vi "Examples.vi"() -> ()   [LabVIEW 2019]
uses:
  <userlib>/MicroPython/VIs/uPythonX/uPythonX.xctl
panel:
  in  "Tab Control":enum32{"Simple", "Page 2"}(tab)
  in  "Driving":T1(xcontrol)={"Port"="130.64.157.92", "All Code"="#!/usr/bin/env pybricks-micropython\n\nfrom pybricks import ev3brick as brick\nfrom pybricks.ev3devices import (Motor, TouchSensor, \n          ColorSensor,InfraredSensor, UltrasonicSensor, GyroSensor)\nfrom pybricks.parameters import (Port, Stop, Direction, Button, Color,\n                                   SoundFile, ImageFile, Align)\nfrom pybricks.tools import print, wait, StopWatch\nfrom pybricks.robotics import DriveBase\nimport time\n\n# plug in\n# A =  left motor\n# D =  right motor\n# \n# S4 =  ultrasonic sensor\n\nleft = Motor(Port.A)\nright = Motor(Port.D)\ndist = UltrasonicSensor(Port.S4)\nwheel_dia = 56\nwheel_spacing = 114\n\ncar = DriveBase(left,right,wheel_dia,wheel_spacing)\ncar.drive_time(speed=20,steering= 90,time = 2000)\nwait(2000)\ncar.drive(20,90)\nwait(200)\ncar.stop(Stop.COAST)  #or COAST, BRAKE, or HOLD\n\nbrick.sound.beep()\nbrick.display.clear()\nwhile not any(brick.buttons()):\n     measured = dist.distance()\n     brick.display.clear()\n     brick.display.text(str(measured),(0,60))\n     if measured < 2000:\n          speed = dist.distance() - 100\n          brick.display.text(str(speed))\n          car.drive(speed,0)\n          wait(10)\n"}
  in  "LED and Sound":T1(xcontrol)={"Port"="130.64.157.92", "All Code"="#!/usr/bin/env pybricks-micropython\n\nfrom pybricks import ev3brick as brick\nfrom pybricks.parameters import Button, Color,ImageFile\nfrom pybricks.tools import print, wait\n\n# A high pitch (1500 Hz) for one second (1000 ms) at 50% volume\nbrick.sound.beep(500, 1000, 20)\n\nwhile True:\n    # Do something if the left button is pressed\n    if Button.LEFT in brick.buttons():\n        print(\"The left button is pressed.\")\n        break\n    wait(100)\nbrick.light(Color.RED)\nLight = [Color.BLACK, Color.GREEN, Color.YELLOW, Color.RED, Color.ORANGE]\n\nfor color in Light:\n    print(color)\n    try:\n        brick.light(color)\n    except:\n        print('bad')\n    wait(500)\n\nbrick.display.clear()\nbrick.display.text(brick.battery.voltage(), (0, 50))\nwhile not Button.CENTER in brick.buttons():\n    wait(100)\nbrick.display.image(ImageFile.UP)\nwhile not Button.CENTER in brick.buttons():\n    wait(100)\n"}
  in  "Sensors":T1(xcontrol)={"Port"="130.64.157.92", "All Code"="#!/usr/bin/env pybricks-micropython\n\nfrom pybricks import ev3brick as brick\nfrom pybricks.ev3devices import (Motor, TouchSensor, \n          ColorSensor,InfraredSensor, UltrasonicSensor, GyroSensor)\nfrom pybricks.parameters import (Port, Stop, Direction, Button, Color,\n                                   SoundFile, ImageFile, Align)\nfrom pybricks.tools import print, wait\n\n# plug in\n# S1 =  touch sensor \n# S2 =  light sensor\n# S3 =  gyro sensor\n# S4 =  ultrasonic sensor\n\ntouch = TouchSensor(Port.S1)\nwhile not touch.pressed():\n     wait (10)\n     \nlight = ColorSensor(Port.S2)\nlight.rgb()\nwait(100)\nlight.color()  \n# returns Color.BLACK, Color.BLUE, Color.GREEN, Color.YELLOW, Color.RED, Color.WHITE, Color.BROWN or None.\nwait(100)\nwhile not (light.color() == Color.YELLOW):\n     wait(100)\nlight.reflection()\nwait(100)\nlight.ambient()\nwait(100)\n\ngyro = GyroSensor(Port.S3)\n\ngyro.reset_angle(0)  # define your starting angle\nwhile gyro.angle() < 90:\n     wait(100)\n     \ngyro.speed()"}
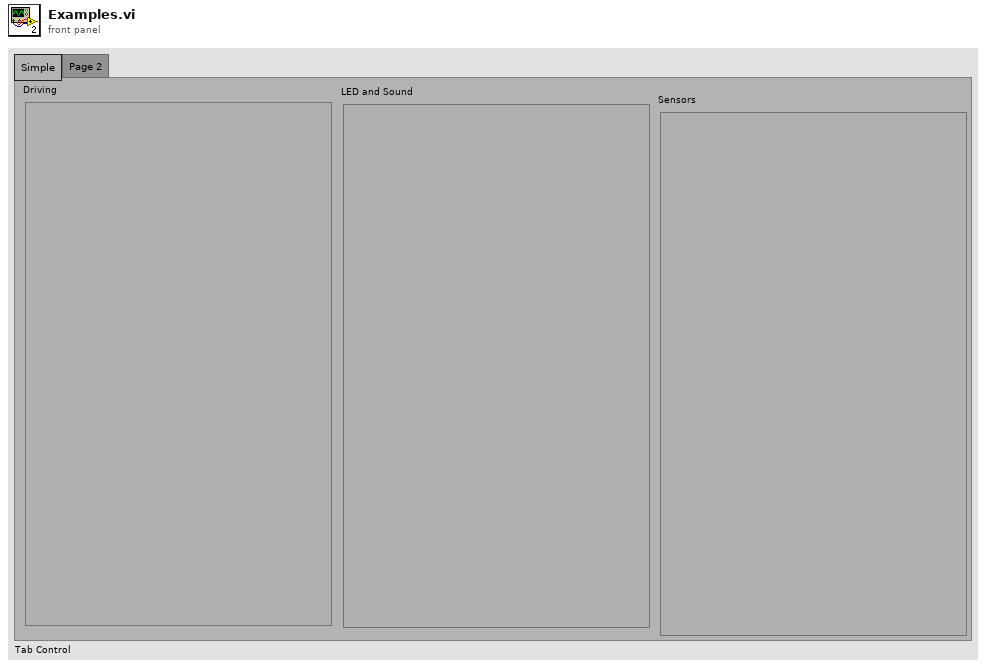
[diagram p1: front panel]
types:
  T1 = cluster{"Port":refnum<visa-resource-name>, "All Code":string}
  T2 = cluster{"VISA Refnum in":refnum<visa-resource-name>, "Python Code":string}
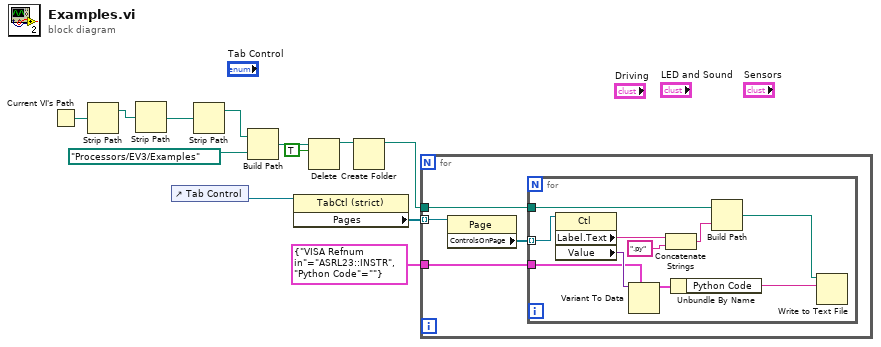
[diagram p0: block diagram]
diagram:
  n1 = Current VI's Path() -> (path=w6:path)
  n2 = Strip Path(path=w6) -> (stripped path=w2:path)  [unwired: 1 out]
  n3 = Strip Path(path=w2) -> (stripped path=w1:path)  [unwired: 1 out]
  n4 = control-ref of="Tab Control"() -> (w3:refnum<vi>)
  n5 = Strip Path(path=w1) -> (stripped path=w7:path)  [unwired: 1 out]
  n6 = Build Path(base path=w7, name or relative path=path "Processors/EV3/Examples") -> (appended path=w10:path)
  n7 = property class="TabCtl (strict)"(reference=w3) -> ("Pages"=w4:refnum<vi>[])  [unwired: 1 in, 2 out]
  n8 = Delete(path (use dialog)=w10, entire hierarchy (F)=TRUE) -> (deleted path=w11:path)  [unwired: 3 in, 2 out]
  n9 = Create Folder(path (use dialog)=w11) -> (created path=w12:path)  [unwired: 2 in, 2 out]
  n10 = for {
    tunnel: w4 -> [w16] mode=indexing
    tunnel: T2 {"VISA Refnum in"="ASRL23::INSTR", "Python Code"=""} ("VOC") -> [w14]
    tunnel: w12 -> [w13]
    n11 = property class="Page"(reference=w16) -> ("ControlsOnPage"=w15:refnum<vi>[])  [unwired: 1 in, 2 out]
    n12 = for {
      tunnel: w15 -> [w26] mode=indexing
      tunnel: w14 -> [w24]
      tunnel: w13 -> [w22]
      n13 = property class="Ctl"(reference=w26) -> ("Label.Text"=w21:string, "Value"=w25:variant)  [unwired: 1 in, 2 out]
      n14 = Variant To Data(type=w24, Variant=w25) -> (data=w23:T2)  [unwired: 1 in, 1 out]
      n15 = Concatenate Strings(w21, ".py" ("string")) -> (w20:string)
      n16 = Unbundle By Name(w23) -> ("Python Code"=w17:string)
      n17 = Build Path(base path=w22, name or relative path=w20) -> (appended path=w18:path)
      n18 = Write to Text File(file (use dialog)=w18, text=w17) -> ()  [unwired: 2 in, 3 out]
    }
  }
